vi "write multiple registers.vi"(8 "error in (no error)":errorcluster, 9 "register values":u16[](array[numeric]) format="%.0x", 10 "addresses":u16[](array[numeric]) format="%.0x", 11 "Stepper in":refnum<class "Stepper.lvclass">) -> (0 "error out":errorcluster, 3 "Stepper out":refnum<class "Stepper.lvclass">)   [LabVIEW 2025, in "Stepper.lvclass"]
uses:
  Stepper.lvclass
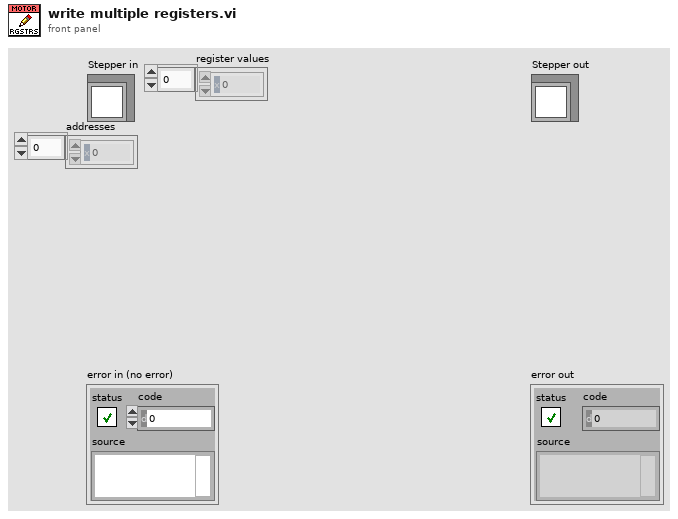
[diagram p1: front panel]
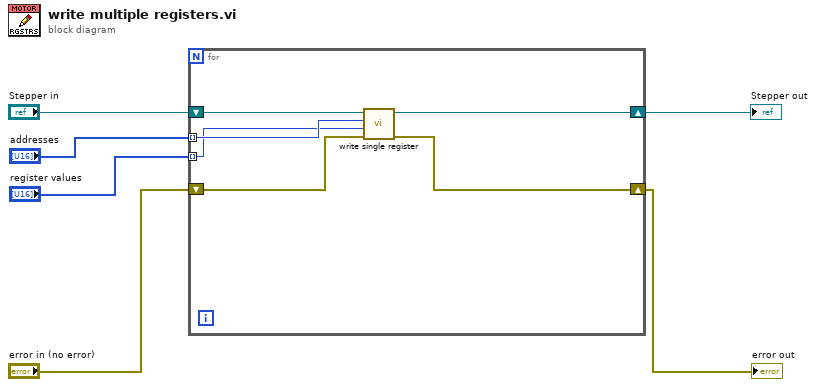
[diagram p0: block diagram]
diagram:
  n1 = for {
    shift-right: [w11] -> w5
    shift-left: "Stepper in" -> [w12]
    shift-right: [w9] -> w3
    shift-left: "error in (no error)" -> [w10]
    tunnel: "addresses" -> [w8] mode=indexing
    tunnel: "register values" -> [w7] mode=indexing
    n2 = call-dynamic "write single register.vi"("error in (no error)"=w10, "register to write"=w7, "address"=w8, "Stepper in"=w12) -> ("error out"=w9:errorcluster, "Stepper out"=w11:refnum<class "Stepper.lvclass">)  [unwired: 6 in]
  }
  "error out" <- w3
  "Stepper out" <- w5
